vi "Large File - create Voltage Current Graphs.vi"(4 "error in (no error)":errorcluster, 7 "tdms file":refnum<k34>) -> (0 "error out":errorcluster, 1 "Full Shot - Discharge Voltage (V) and Current (A) against Time (s)":waveform(dbl)[](graph), 3 "tdms file out":refnum<k34>)   [LabVIEW 2015]
uses:
  <vilib>/Waveform/WDTOps.llb/WDT Get Waveform Subset DBL.vi
  <vilib>/measure/maresamp.llb/Resample Waveform (continuous).vi
  <vilib>/Waveform/WDTOps.llb/WDT Append Waveforms DBL.vi
  <vilib>/Analysis/NI_AAL_SigProc.lvlib
  <vilib>/measure/NI_MAPro.lvlib
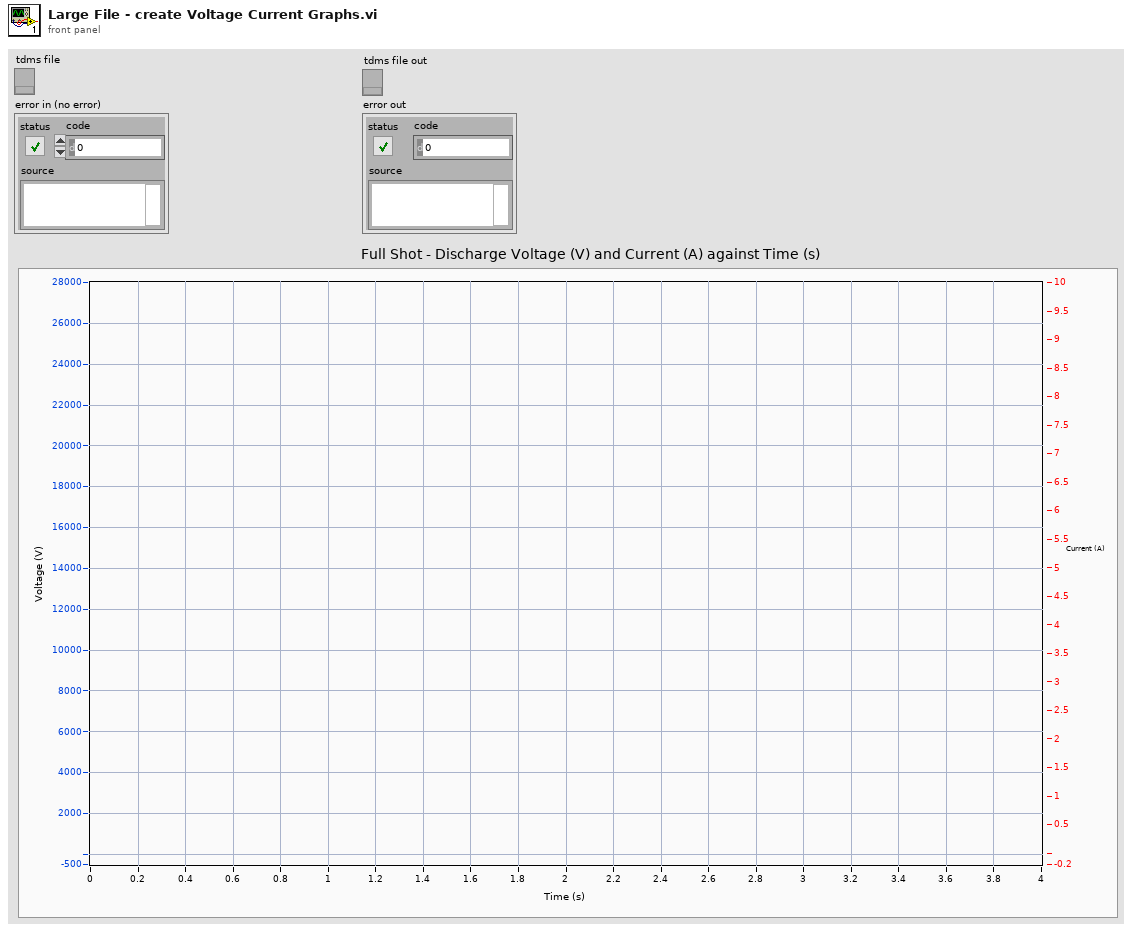
[diagram p1: front panel]
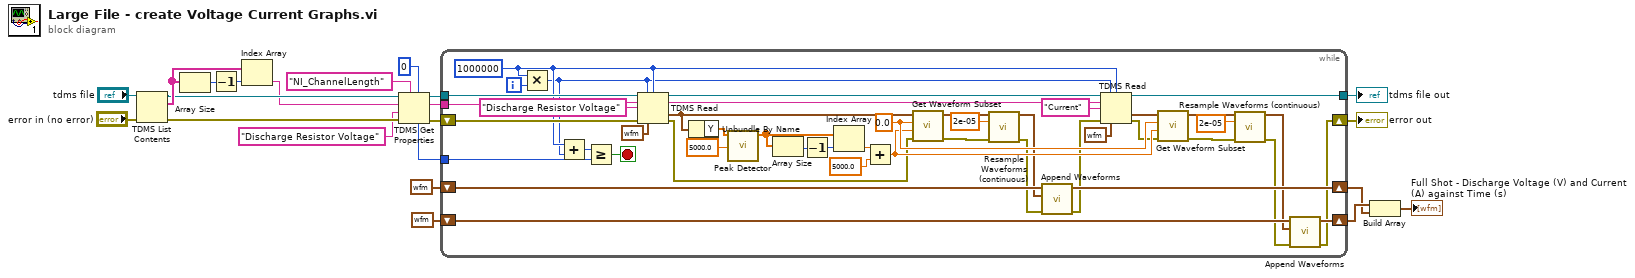
[diagram p0: block diagram]
diagram:
  n1 = TDMS List Contents(4:"error in (no error)", 7:"tdms file") -> (0:w10:errorcluster, 2:w20:string[], 3:w9:refnum<k34>)  [unwired: 1 in, 1 out]
  n2 = Array Size(array=w20) -> (size(s)=w22:i32)
  n3 = Decrement(x=w22) -> (x-1=w21:i32)
  n4 = Index Array(array=w20, index=w21) -> (element=w8:string)
  n5 = TDMS Get Properties(5:0, 7:"NI_ChannelLength" ("property name"), 8:w10, 9:"Discharge Resistor Voltage" ("group name in"), 10:w8, 11:w9) -> (0:w11:errorcluster, 2:w6:string, 3:w12:refnum<k34>, 4:w7:i32)  [unwired: 2 out]
  n6 = while {
    tunnel: w6 -> [w24]
    shift-right: [w48] -> w17
    shift-left: waveform(dbl) {"t0"=timestamp(0 s since 1904-01-01), "dt"=4e-05, "Y"=[]} ("waveform out") -> [w47]
    tunnel: w12 -> [w61]
    tunnel: [w30] -> w2
    shift-right: [w25] -> w1
    shift-left: w11 -> [w62]
    shift-right: [w46] -> w16
    shift-left: waveform(dbl) {"t0"=timestamp(0 s since 1904-01-01), "dt"=4e-05, "Y"=[]} ("waveform out") -> [w45]
    tunnel: w7 -> [w42]
    i -> [w44]
    stop <- w33 stop-if-true
    w41 = i64 1000000
    w52 = 0.0 ("start samples/time")
    n7 = Multiply(x=w41, y=w44) -> (x*y=w40:i64)
    n8 = Add(x=w41, y=w40) -> (x+y=w43:i64)
    n9 = Greater Or Equal?(x=w43, y=w42) -> (x >= y?=w33:bool)
    n10 = TDMS Read(0:w61, 1:w40, 2:w41, 5:w24, 7:"Discharge Resistor Voltage" ("group name in"), 11:w62, 12:waveform(dbl) {"t0"=timestamp(0 s since 1904-01-01), "dt"=1.0, "Y"=[]} ("Waveform")) -> (4:w65:refnum<k34>, 6:w23:string, 10:w58:waveform(dbl), 15:w50:errorcluster)  [unwired: 1 in, 2 out]
    n11 = Unbundle By Name(w58) -> ("Y"=w60:dbl[])
    n12 = call <vilib>:"Peak Detector.vi"("threshold"=5000.0, "X"=w60) -> ("Locations"=w32:dbl[])  [unwired: 5 in, 4 out]
    n13 = Array Size(array=w32) -> (size(s)=w57:i32)
    n14 = Decrement(x=w57) -> (x-1=w56:i32)
    n15 = Index Array(array=w32, index=w56) -> (element=w55:dbl)
    n16 = Add(x=w55, y=5000.0) -> (x+y=w51:dbl)
    n17 = call-poly <vilib>:"Get Waveform Subset.vi"("error in (no error)"=w50, "duration"=w51, "start samples/time"=w52, "waveform in"=w58) -> ("error out"=w29:errorcluster, "waveform out"=w39:waveform(dbl))  [unwired: 2 in, 2 out]
    n18 = call-poly <vilib>:"Resample Waveforms (continuous).vi"("waveform in"=w39, "dt"=2e-05, "error in (no error)"=w29) -> ("resampled waveform out"=w38:waveform(dbl), "error out"=w28:errorcluster)  [unwired: 8 in, 3 out]
    n19 = call-poly <vilib>:"Append Waveforms.vi"("error in (no error)"=w28, "waveform B"=w38, "waveform A"=w45) -> ("error out"=w27:errorcluster, "waveform out"=w46:waveform(dbl))  [unwired: 7 in]
    n20 = TDMS Read(0:w65, 1:w40, 2:w41, 5:w23, 7:"Current" ("group name in"), 11:w27, 12:waveform(dbl) {"t0"=timestamp(0 s since 1904-01-01), "dt"=1.0, "Y"=[]} ("Waveform")) -> (4:w30:refnum<k34>, 10:w53:waveform(dbl), 15:w49:errorcluster)  [unwired: 1 in, 3 out]
    n21 = call-poly <vilib>:"Get Waveform Subset.vi"("error in (no error)"=w49, "duration"=w51, "start samples/time"=w52, "waveform in"=w53) -> ("error out"=w31:errorcluster, "waveform out"=w37:waveform(dbl))  [unwired: 2 in, 2 out]
    n22 = call-poly <vilib>:"Resample Waveforms (continuous).vi"("waveform in"=w37, "dt"=2e-05, "error in (no error)"=w31) -> ("resampled waveform out"=w36:waveform(dbl), "error out"=w26:errorcluster)  [unwired: 8 in, 3 out]
    n23 = call-poly <vilib>:"Append Waveforms.vi"("error in (no error)"=w26, "waveform B"=w36, "waveform A"=w47) -> ("error out"=w25:errorcluster, "waveform out"=w48:waveform(dbl))  [unwired: 7 in]
  }
  "tdms file out" <- w2
  "error out" <- w1
  n24 = Build Array(w17, w16) -> (→"Full Shot - Discharge Voltage (V) and Current (A) against Time (s)":waveform(dbl)[])
